vi "ROS_Topic_Write_Continuous_Primitive.vi"(2 "Msg in":string, 3 "ROS in":T1={"topic port"=0, "Node"="", "topic"="", "type"="", "node port"=0, "error "={"status"=FALSE, "code"=0, "source"=""}, "Direction"=enum."Node", "APIs"=[], "Update (ms)"=1, "write queue"=1}) -> (1 "ROS out":T1={"topic port"=0, "Node"="", "topic"="", "type"="", "node port"=0, "error "={"status"=FALSE, "code"=0, "source"=""}, "Direction"=enum."Node", "APIs"=[], "Update (ms)"=1, "write queue"=1})   [LabVIEW 2010]
doc: "Instructs the server to write out the data as often as possible. The server updates the message being sent upon a new ROS_Topic_Write call."
uses:
  <userlib>/ROSforLV/ROS/Code/SubVIs/_ROSControl.ctl
  <userlib>/ROSforLV/ROS/Code/SubVIs/_ROSDirection.ctl
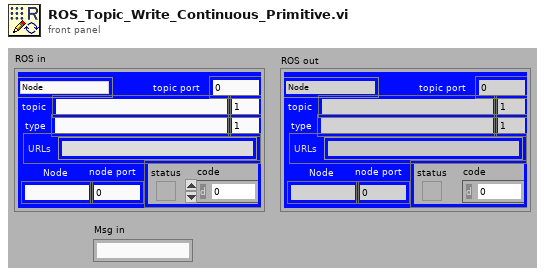
[diagram p1: front panel]
types:
  T1 = typedef "_ROSControl.ctl" = cluster{"topic port":u16, "Node":string, "topic":string, "type":string, "node port":u32, "error ":errorcluster, "Direction":T2, "APIs":string[], "Update (ms)":u16, "write queue":u16}
  T2 = typedef "_ROSDirection.ctl" = enum16{"Node", "Publisher", "Subscriber", "Service Client"}
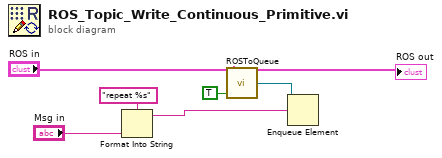
[diagram p0: block diagram]
diagram:
  n1 = Format Into String(format string="repeat %s" ("name (unnamed)"), "Msg in") -> (resulting string=w4:string)  [unwired: 2 in, 1 out]
  n2 = call <userlib>:"ROSToQueue.vi"("Wait?"=TRUE, "ROS"="ROS in") -> ("queue"=w2:refnum<queue>)  [unwired: 2 in, 1 out]
  n3 = Enqueue Element(queue=w2, element=w4) -> ()  [unwired: 2 in, 3 out]
  "ROS out" <- "ROS in"
